vi "Reset.vi"(8 "error in (no error)":errorcluster, 11 "PEU in":refnum<class "PEU.lvclass">) -> (0 "error out":errorcluster, 3 "PEU out":refnum<class "PEU.lvclass">)   [LabVIEW 2020, in "PEU.lvlib" / "PEU.lvclass"]
uses:
  PEU.lvclass
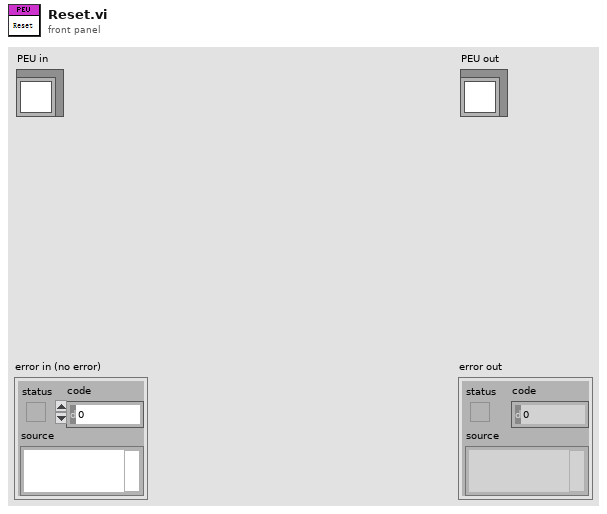
[diagram p1: front panel]
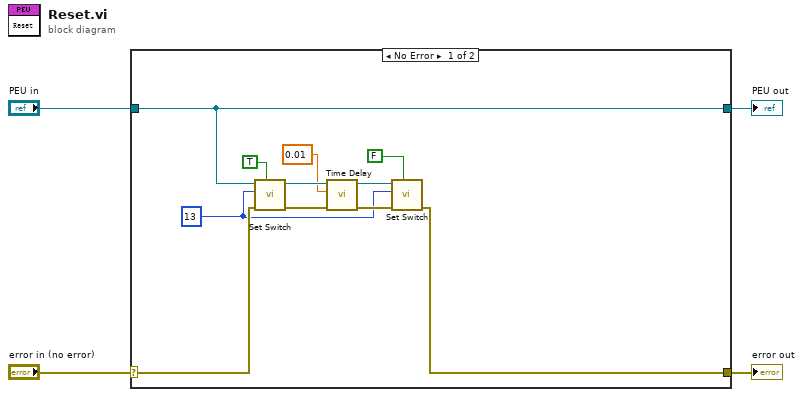
[diagram p0: block diagram]
diagram:
  n1 = case shown="No Error" "error in (no error)" {
    selector: "error in (no error)" -> [w7 w16]
    tunnel: [w6 w16] -> w3
    tunnel: [w9 w15] -> w1
    tunnel: "PEU in" -> [w9 w15]
    frame No Error {
      w5 = u16 13 ("Pin")
      n2 = call "Set Switch.vi"("ON/OFF"=TRUE, "error in (no error)"=w7, "Pin"=w5, "PEU in"=w9) -> ("error out"=w13:errorcluster, "PEU out"=w11:refnum<class "PEU.lvclass">)  [unwired: 6 in]
      n3 = call "Time Delay"("error in (no error)"=w13, "Delay Time (s)"=0.01) -> ("error out"=w12:errorcluster)  [unwired: 9 in]
      n4 = call "Set Switch.vi"("ON/OFF"=FALSE, "error in (no error)"=w12, "Pin"=w5, "PEU in"=w11) -> ("error out"=w6:errorcluster)  [unwired: 6 in, 1 out]
    }
    frame Error {
    }
  }
  "error out" <- w3
  "PEU out" <- w1
